vi "thermo_interpolate_correction.vi"(3 "input":dbl, 5 "temp cor":dbl[][](array[numeric]) caption="corrections" format="%.1f") -> (0 "output":dbl, 1 "out of range":bool, 2 "fail":bool)   [LabVIEW 2020]
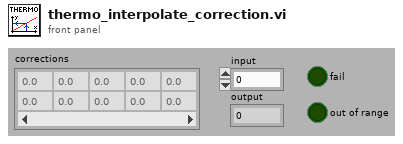
[diagram p1: front panel]
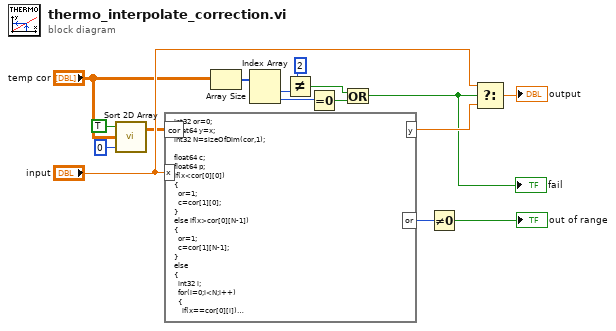
[diagram p0: block diagram]
diagram:
  n1 = call "Sort 2D Array.vi"("Sort By (Column:F)"=TRUE, "Unsorted 2D Array"="temp cor", "Column/Row to Sort By"=u32 0) -> ("Sorted 2D Array"=w4:dbl[][])  [unwired: 2 in, 1 out]
  n2 = formula code="int32 or=0;\nfloat64 y=x;\nint32 N=sizeOfDim(cor,1);\n\nfloat64 c;\nfloat64 p;\nif(x<cor[0][0])\n{\n  or=1;\n  c=cor[1][0];\n}\nelse if(x>cor[0][N-1])\n{\n  or=1;\n  c=cor[1][N-1];\n}\nelse\n{\n  int32 i;\n  for(i=0;i<N;i++)\n  {\n    if(x==cor[0][i])\n    {\n      c=cor[1][i];\n      break;\n    }\n    else if(x<cor[0][i])\n    {\n      p=(x - cor[0][i-1])/(cor[0][i] - cor[0][i-1]);\n      c=cor[1][i]*p + cor[1][i-1]*(1-p);\n      break;\n    }\n  }\n}\ny=x+c;"("cor"=w4, "x"="input") -> ("y"=w8:dbl, "or"=w7:i32)
  n3 = Array Size(array="temp cor") -> (size(s)=w16:i32[])
  n4 = Index Array(array=w16) -> (element #1=w15:i32, element #2=w13:i32)  [unwired: 2 in]
  n5 = Not Equal?(x=2, y=w15) -> (x != y?=w11:bool)
  n6 = Equal To 0?(x=w13) -> (x = 0?=w12:bool)
  n7 = Or(x=w11, y=w12) -> (x .or. y?=w1:bool)
  "fail" <- w1
  n8 = Not Equal To 0?(x=w7) -> (x != 0?=→"out of range":bool)
  n9 = Select(t="input", s=w1, f=w8) -> (s? t:f=→"output":dbl)
